vi "cblas zsymm.vi"(0 "A":T4, 1 "B":T4, 2 "C":T4, 3 "alpha":cdb=1.0+0.0i, 4 "beta":cdb=1.0+0.0i, 5 "order":T3=101 items=["CblasRowMajor"=101, "CblasColMajor"=102], 7 "uplo":T1=121 items=["CblasUpper"=121, "CblasLower"=122], 8 "lda":i32, 9 "m":i32=-1, 10 "ldb":i32, 11 "n":i32=-1, 12 "ldc":i32, 13 "side":T2=141 items=["CblasLeft"=141, "CblasRight"=142]) -> (14 "zsymm":T4, 19 "error":i32)   [LabVIEW 2024, in "NI_AALBLAS.lvlib"]
uses:
  NI_AALBLAS.lvlib
  ComplexMatrix.ctl
  Order.ctl
  Side.ctl
  UpLo.ctl
  NI_Matrix.lvlib
  <resource>/lvblas.dll
panel:
  # "void cblas_zsymm(order, side, uplo, m, n, *alpha,*A, lda, *B, ldb, *beta, *C, ldc)"
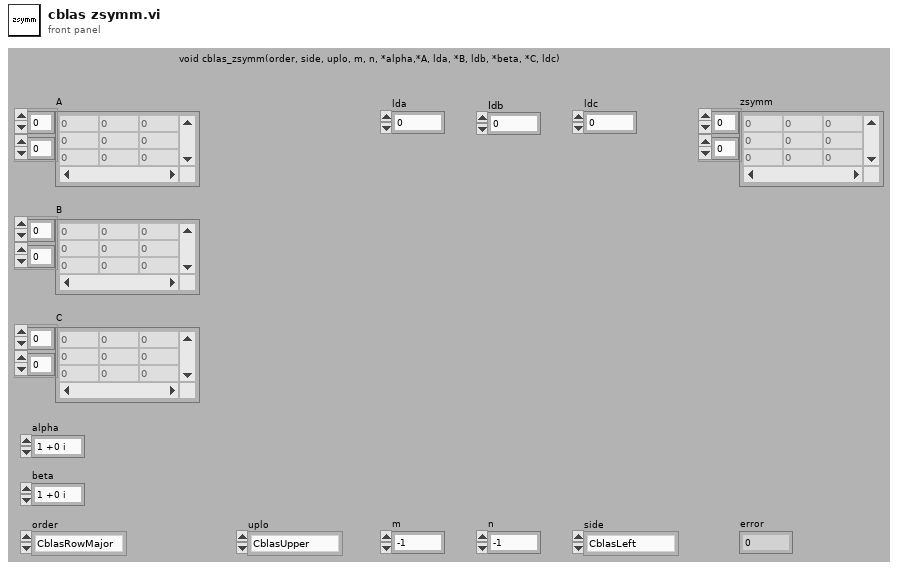
[diagram p1: front panel]
types:
  T1 = typedef "NI_AALBLAS.lvlib/UpLo.ctl" = i32
  T2 = typedef "NI_AALBLAS.lvlib/Side.ctl" = i32
  T3 = typedef "NI_AALBLAS.lvlib/Order.ctl" = i32
  T4 = typedef "NI_Matrix.lvlib/ComplexMatrix.ctl" = cdb[][]
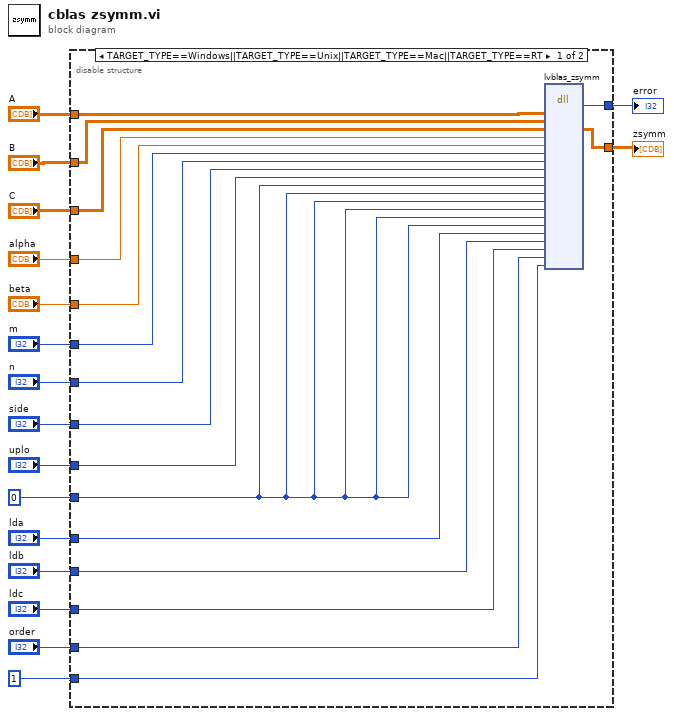
[diagram p0: block diagram]
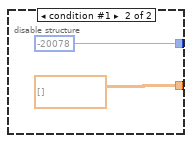
[diagram p2: hidden frame]
diagram:
  n1 = disable-structure shown="TARGET_TYPE==Windows||TARGET_TYPE==Unix||TARGET_TYPE==Mac||TARGET_TYPE==RT" {
    disable-tunnel: [w34 -20078 ("error")] -> w17
    disable-tunnel: "A" -> [w33 _]
    disable-tunnel: "B" -> [w32 _]
    disable-tunnel: "C" -> [w31 _]
    disable-tunnel: "alpha" -> [w30 _]
    disable-tunnel: "beta" -> [w29 _]
    disable-tunnel: [w28 T4 [] ("Complex Matrix")] -> w16
    disable-tunnel: "side" -> [w27 _]
    disable-tunnel: "uplo" -> [w26 _]
    disable-tunnel: 0 -> [w25 _]
    disable-tunnel: "order" -> [w24 _]
    disable-tunnel: "m" -> [w23 _]
    disable-tunnel: "n" -> [w22 _]
    disable-tunnel: "lda" -> [w21 _]
    disable-tunnel: "ldb" -> [w20 _]
    disable-tunnel: "ldc" -> [w19 _]
    disable-tunnel: 1 -> [w18 _]
    frame condition #0 (active) {
      n2 = dll-call lib="C:/Program Files (x86)/National Instruments/LabVIEW 2024/resource/lvblas.*" fn="lvblas_zsymm" ("CBLAS.dll:MtrxxMtrxH")("A"=w33, "B"=w32, "C"=w31, "alpha"=w30, "beta"=w29, "m"=w23, "n"=w22, "side"=w27, "uplo"=w26, "startARow"=w25, "startACol"=w25, "startBRow"=w25, "startBCol"=w25, "startCRow"=w25, "startCCol"=w25, "lda"=w21, "ldb"=w20, "ldc"=w19, "order"=w24, "check"=w18) -> ("error"=w34:i32, "C"=w28:T4)  [unwired: 22 in, 2 out]
    }
    frame condition #1 {
    }
  }
  "zsymm" <- w16
  "error" <- w17
